vi "VDH-cancelCalibration.vi"(8 "error in (no error)":errorcluster, 11 "VDH-VNA_data_handler in":refnum<class "VDH-VNA_data_handler.lvclass">) -> (0 "error out":errorcluster, 3 "VDH-VNA_data_handler out":refnum<class "VDH-VNA_data_handler.lvclass">)   [LabVIEW 2020, in "VDH-VNA_data_handler.lvlib" / "VDH-VNA_data_handler.lvclass"]
uses:
  VDH-VNA_data_handler.lvclass
  VDH-VNA_data_handler.lvclass/VDH-VNA_data_handler.ctl
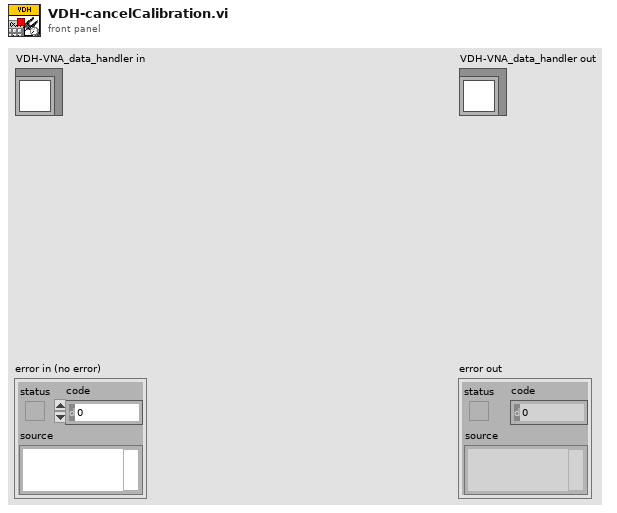
[diagram p1: front panel]
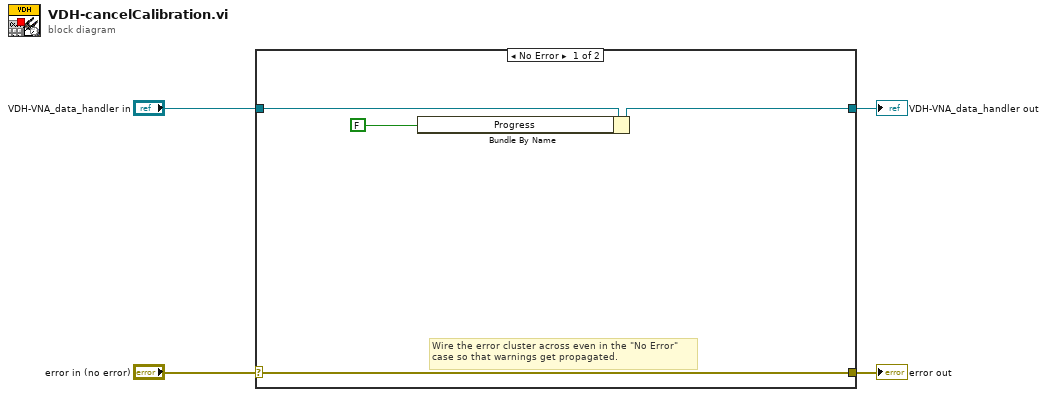
[diagram p0: block diagram]
diagram:
  n1 = case shown="No Error" "error in (no error)" {
    selector: "error in (no error)" -> [w7 w10]
    tunnel: [w7 w10] -> w3
    tunnel: [w6 w9] -> w1
    tunnel: "VDH-VNA_data_handler in" -> [w8 w9]
    frame No Error {
      # "Wire the error cluster across even in the \"No Error\"\ncase so that warnings get propagated."
      n2 = Bundle By Name(cluster=w8, "Progress"=FALSE ("Calibration Status.Calib In Progress")) -> (w6:refnum<class "VDH-VNA_data_handler.lvclass">)
    }
    frame Error {
    }
  }
  "error out" <- w3
  "VDH-VNA_data_handler out" <- w1
